vi "Run Core.vi"(8 "Error In":errorcluster, 9 "Timeout (s)":dbl, 10 "Meas In":refnum<class "LogError.lvclass">, 11 "Logger In":refnum<class "ILogger.lvclass">) -> (0 "Error Out":errorcluster, 1 "Timeout?":bool, 2 "Result Out":refnum<class "IResult.lvclass">, 3 "Logger Out":refnum<class "ILogger.lvclass">)   [LabVIEW 2020, in "LogError.lvclass"]
uses:
  LogError.lvclass
  LogMessage/AbstractLogMessage.lvclass
  ILogger/ILogger.lvclass
  C:/Repo/LabVIEW-SOLID-Examples/Template-Logger/LogMessage/LogMessage.lvclass
  C:/Repo/LabVIEW-SOLID-Examples/Template-Logger/IAction/IAction.lvclass
  C:/Repo/LabVIEW-SOLID-Examples/Template-Logger/IValid/IValid.lvclass
  C:/Repo/LabVIEW-SOLID-Examples/Template-Logger/LogError/LogError.lvclass
  IResult/IResult.lvclass
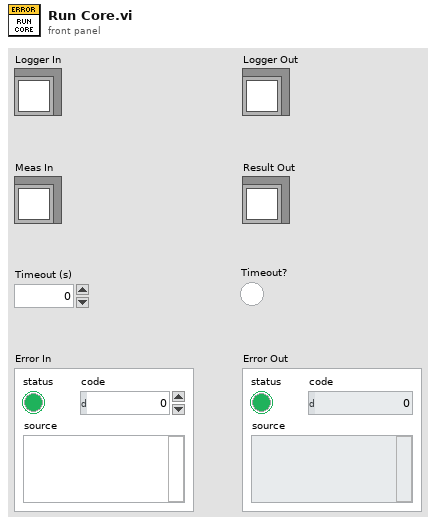
[diagram p1: front panel]
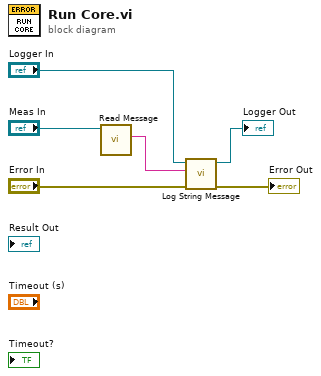
[diagram p0: block diagram]
diagram:
  n1 = call "Read Message.vi"("LogMessage In"="Meas In") -> ("Message"=w2:string)  [unwired: 9 in, 1 out]
  n2 = call-dynamic "Log String Message.vi"("Error In"="Error In", "Message"=w2, "ILogger In"="Logger In") -> ("Error Out"=→"Error Out":errorcluster, "ILogger Out"=→"Logger Out":refnum<class "ILogger.lvclass">)  [unwired: 7 in]
